vi "Hardware Device Get All Info.vi"(8 "error in":errorcluster, 11 "NI Analog Output in":refnum<class "NI Analog Output.lvclass">) -> (0 "error out":errorcluster, 3 "NI Analog Output out":refnum<class "NI Analog Output.lvclass">)   [LabVIEW 2023, in "HardwareAbstractionLayer_LVOOP.lvlib" / "NI Analog Output.lvclass"]
doc: "This VI Device Physical Channel Read"
uses:
  NI Analog Output.lvclass
  NI Analog Output.lvclass/NI Analog Output.ctl
  <resource>/objmgr/daqmx.rc
panel:
  out "AO.PhysicalChans":tag[](array[tag])
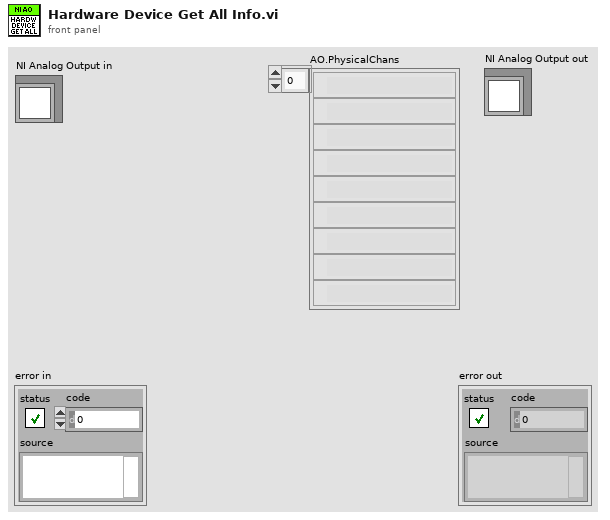
[diagram p1: front panel]
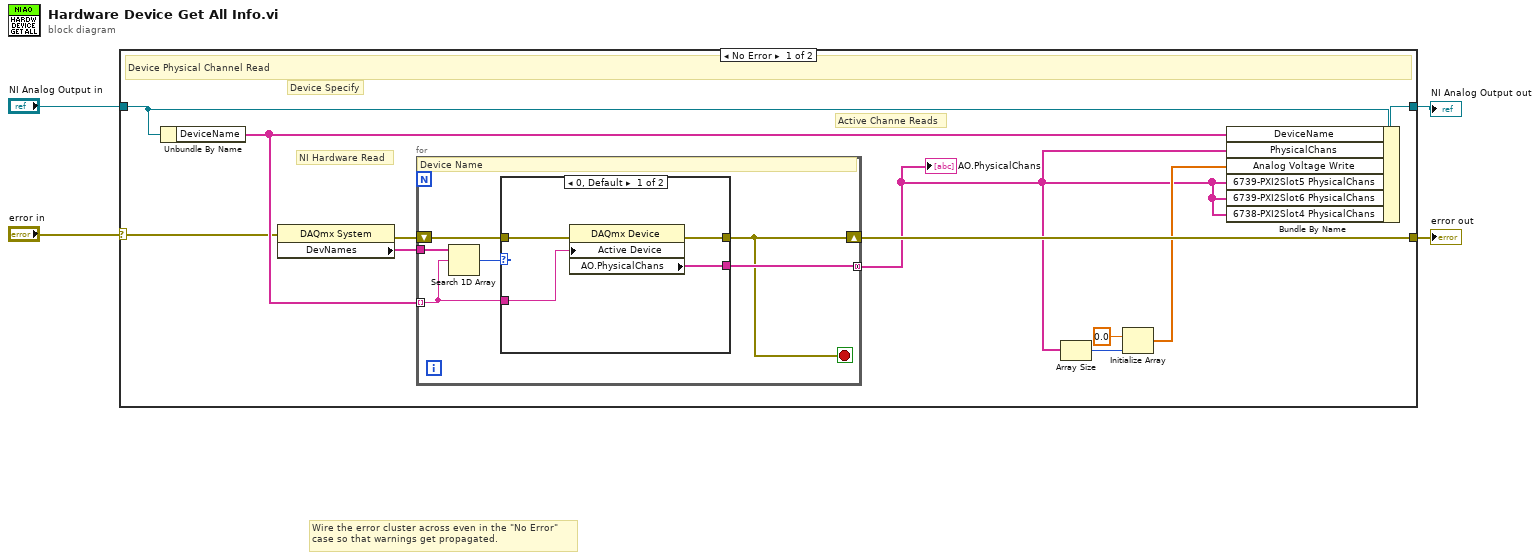
[diagram p0: block diagram]
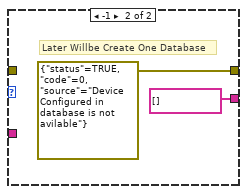
[diagram p2: hidden frame]
diagram:
  # "Wire the error cluster across even in the \"No Error\"\ncase so that warnings get propagated."
  n1 = case shown="No Error" "error in" {
    selector: "error in" -> [w6 w29]
    tunnel: [w8 w29] -> w3
    tunnel: [w12 w28] -> w1
    tunnel: "NI Analog Output in" -> [w11 w28]
    frame No Error {
      # "Active Channe Reads"
      # "Device Specify"
      # "NI Hardware Read"
      # "Device Physical Channel Read"
      n2 = Unbundle By Name(w11) -> ("DeviceName"=w15:tag[])
      n3 = property class="DAQmx System"(error in=w6) -> (error out=w13:errorcluster, "DevNames"=w14:tag[])  [unwired: 1 in, 1 out]
      n4 = for {
        tunnel: w15 -> [w18] mode=indexing
        tunnel: w14 -> [w19]
        tunnel: [w17] -> w5 mode=concatenating
        shift-right: [w16] -> w8
        shift-left: w13 -> [w20]
        stop <- w16 stop-if-true
        # "Device Name"
        n5 = Search 1D Array(1D array=w19, element=w18) -> (index of element=w21:i32)  [unwired: 1 in]
        n6 = case shown="0, Default" w21 {
          tunnel: w20 -> [w23 _]
          tunnel: [w22 errorcluster {"status"=TRUE, "code"=0, "source"="Device  Configured in database is not avilable"} ("error out")] -> w16
          tunnel: w18 -> [w25 _]
          tunnel: [w24 tag[] [] ("AI.PhysicalChans")] -> w17
          frame 0, Default {
            n7 = property class="DAQmx Device"(error in=w23, "Active Device"=w25) -> (error out=w22:errorcluster, "AO.PhysicalChans"=w24:tag[])  [unwired: 1 in, 1 out]
          }
          frame -1 {
            # "Later Willbe Create One Database"
          }
        }
      }
      "AO.PhysicalChans" <- w5
      n8 = Array Size(array=w5) -> (size(s)=w10:i32)
      n9 = Initialize Array(0.0, w10) -> (w7:dbl[])
      n10 = Bundle By Name(cluster=w11, "DeviceName"=w15, "PhysicalChans"=w5, "Analog Voltage Write"=w7, "6739-PXI2Slot5 PhysicalChans"=w5, "6739-PXI2Slot6 PhysicalChans"=w5, "6738-PXI2Slot4 PhysicalChans"=w5) -> (w12:refnum<class "NI Analog Output.lvclass">)
    }
    frame Error {
    }
  }
  "error out" <- w3
  "NI Analog Output out" <- w1
